vi "Write Column Header Strings[].vi"(8 "error in (no error)":errorcluster, 10 "ColHdrs[]":string[](array[string]), 11 "AdjustableMulticolumnListbox.lvclass in":refnum<class "AdjMCLB.lvclass">) -> (0 "error out":errorcluster, 3 "AdjustableMulticolumnListbox.lvclass out":refnum<class "AdjMCLB.lvclass">)   [LabVIEW 2020, in "AdjMCLB.lvclass"]
uses:
  AdjMCLB.lvclass
  <vilib>/QSI/QControls/QControl Classes/MulticolumnListbox/MulticolumnListbox.lvclass
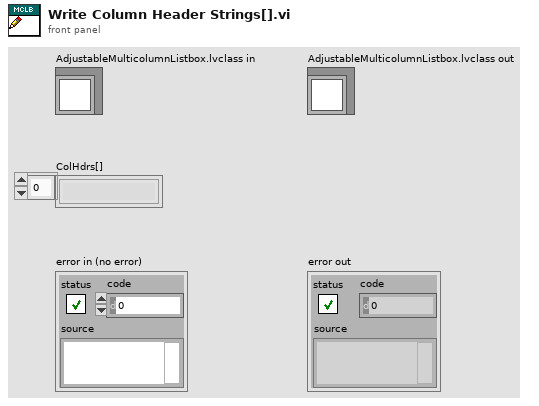
[diagram p1: front panel]
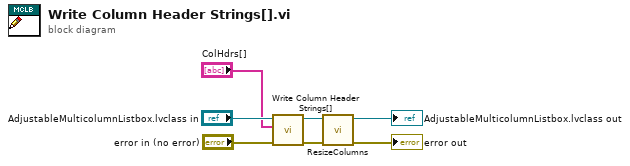
[diagram p0: block diagram]
diagram:
  n1 = call-parent "Write Column Header Strings[].vi"("error in (no error)"="error in (no error)", "ColHdrs[]"="ColHdrs[]", "MulticolumnListbox.lvclass in"="AdjustableMulticolumnListbox.lvclass in") -> ("error out"=w1:errorcluster, "MulticolumnListbox.lvclass out"=w4:refnum<class "AdjMCLB.lvclass">)  [unwired: 7 in]
  n2 = call "ResizeColumns.vi"("error in (no error)"=w1, "AdjustableMulticolumnListbox in"=w4) -> ("error out"=→"error out":errorcluster, "AdjustableMulticolumnListbox out"=→"AdjustableMulticolumnListbox.lvclass out":refnum<class "AdjMCLB.lvclass">)  [unwired: 8 in]
